vi "Make Initial Guess.vi"(8 "error in (no error)":errorcluster, 10 "Desired Field":dbl, 11 "Magna Power in":refnum<class "Magna Power.lvclass">) -> (0 "error out":errorcluster, 2 "First guess":dbl, 3 "Magna Power out":refnum<class "Magna Power.lvclass">)   [LabVIEW 2012, in "Magna Power.lvclass"]
uses:
  Magna Power.lvclass
  Magna Power.lvclass/Magna Power.ctl
  Magna Power Constants.vi
  <vilib>/gmath/NI_Gmath.lvlib
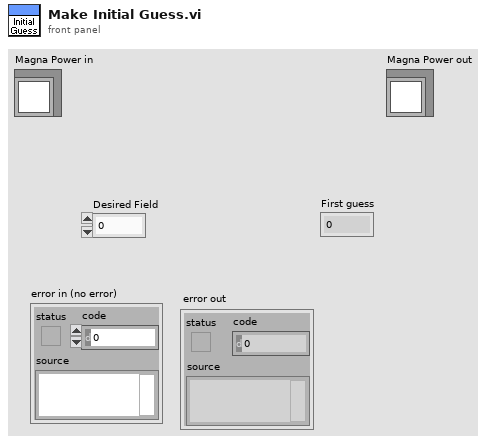
[diagram p1: front panel]
types:
  T1 = cluster{"Magna Current":dbl[], "Magnetic Field":dbl[], "Fluke Voltage":dbl[]}
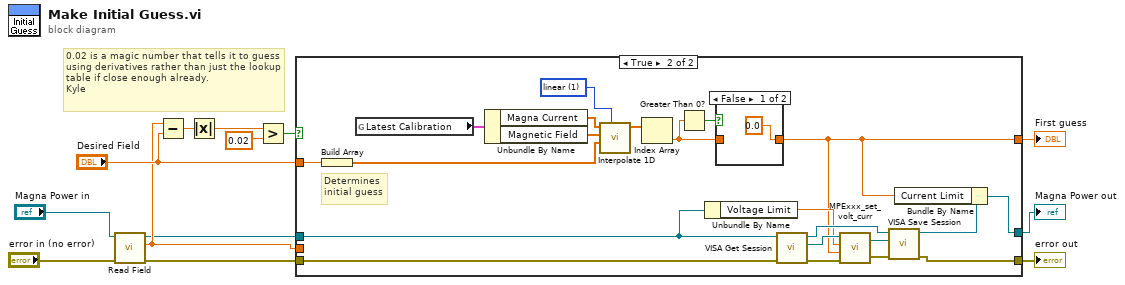
[diagram p0: block diagram]
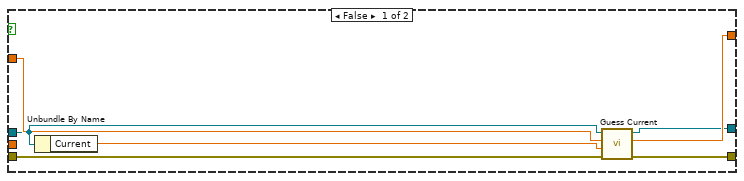
[diagram p2: hidden frame]
diagram:
  # "0.02 is a magic number that tells it to guess using derivatives rather than just the lookup table if close enough already.\nKyle"
  n1 = call "Read Field.vi"("error in (no error)"="error in (no error)", "Magna Power in"="Magna Power in") -> ("error out"=w3:errorcluster, "Field (T)"=w6:dbl, "Magna Power out"=w4:refnum<class "Magna Power.lvclass">)  [unwired: 7 in]
  n2 = Subtract(x=w6, y="Desired Field") -> (x-y=w12:dbl)
  n3 = Absolute Value(x=w12) -> (abs(x)=w11:dbl)
  n4 = Greater?(x=w11, y=0.02) -> (0:w9:bool)
  n5 = case shown="True" w9 {
    tunnel: w3 -> [w16 w32]
    tunnel: "Desired Field" -> [w20 w33]
    tunnel: [w19 w22] -> w7
    tunnel: w4 -> [w18 w25]
    tunnel: w6 -> [_ _]
    tunnel: [w15 w26] -> w2
    tunnel: [w14 w21] -> w1
    frame False {
      n6 = Unbundle By Name(w18) -> ("Current"=w17:dbl)
      n7 = call "Guess Current.vi"("error in (no error)"=w16, "Current guess"=w17, "Desired Field"=w20, "Magna Power in"=w18) -> ("error out"=w15:errorcluster, "New guess"=w19:dbl, "Magna Power out"=w14:refnum<class "Magna Power.lvclass">)  [unwired: 4 in, 1 out]
    }
    frame True {
      w40 = 1 items=["nearest", "linear", "spline", "cubic Hermite", "Lagrange"] ("method")
      # "Determines\ninitial guess"
      n8 = Build Array(w33) -> (w39:dbl[])
      n9 = global read "Magna Power Constants.vi" "Latest Calibration"() -> (w41:T1)
      n10 = Unbundle By Name(w41) -> ("Magna Current"=w36:dbl[], "Magnetic Field"=w37:dbl[])
      n11 = call <vilib>:"Interpolate 1D.vi"("method"=w40, "xi"=w39, "X"=w37, "Y"=w36) -> ("yi"=w38:dbl[])  [unwired: 5 in, 2 out]
      n12 = Index Array(array=w38) -> (element=w34:dbl)  [unwired: 1 in]
      n13 = Greater Than 0?(x=w34) -> (x > 0?=w35:bool)
      n14 = Unbundle By Name(w25) -> ("Voltage Limit"=w24:dbl)
      n15 = case shown="False" w35 {
        tunnel: [0.0 ("Numeric") w43] -> w22
        tunnel: w34 -> [_ w43]
        frame False {
        }
        frame True {
        }
      }
      n16 = call-dynamic "VISA Get Session.vi"("error in (no error)"=w32, "Instrument.lvclass in"=w25) -> ("error out"=w31:errorcluster, "VISA Resource Name"=w30:refnum<visa-resource-name>, "Instrument.lvclass out"=w27:refnum<class "Magna Power.lvclass">)  [unwired: 6 in, 1 out]
      n17 = call "MPExxx_set_volt_curr.vi"("error in (no error)"=w31, "Set Current"=w22, "Set Voltage"=w24, "VISA session"=w30) -> ("error out"=w28:errorcluster, "dup VISA session"=w29:refnum<visa-resource-name>)
      n18 = call-dynamic "VISA Save Session.vi"("error in (no error)"=w28, "VISA Resource Name"=w29, "Instrument.lvclass in"=w27) -> ("error out"=w26:errorcluster, "Instrument.lvclass out"=w23:refnum<class "Magna Power.lvclass">)  [unwired: 7 in]
      n19 = Bundle By Name(cluster=w23, "Current Limit"=w22) -> (w21:refnum<class "Magna Power.lvclass">)
    }
  }
  "First guess" <- w7
  "error out" <- w2
  "Magna Power out" <- w1
